vi "Previous Button Facade.vi"(0 "Data In":T4, 2 "Display State In":T2, 3 "Container State":T3) -> (6 "Data Out":T4, 7 "Display State Out":T2, 8 "Action":T1)   [LabVIEW 2010, in "Previous Button (System).xctl"]
uses:
  <vilib>/Navigation Controls/Previous Button System/Previous Button (System).xctl
  <vilib>/Navigation Controls/Previous Button System/Previous Button Data.ctl
  <vilib>/_xctls/Container State.ctl
  <vilib>/Navigation Controls/Previous Button System/Previous Button State.ctl
  <vilib>/_xctls/Action.ctl
  <vilib>/_xctls/XControlSupport.lvlib
  <vilib>/Navigation Controls/NI_Navigation.lvlib
panel:
  out "Error":bool
  in  "Prev Button":bool
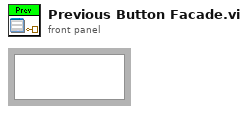
[diagram p1: front panel]
types:
  T1 = typedef "XControlSupport.lvlib/Action.ctl" = cluster{"Data Changed?":bool, "State Changed?":bool, "Action Name":string}
  T2 = typedef "Previous Button (System).xctl/Previous Button State.ctl" = cluster{"Button Text":string}
  T3 = typedef "XControlSupport.lvlib/Container State.ctl" = cluster{"Indicator?":bool, "Run Mode?":bool, " Refnum":refnum<vi>}
  T4 = typedef "Previous Button (System).xctl/Previous Button Data.ctl" = bool
  T5 = enum32{"Invalid", "Standard", "Closed", "Hidden", "Minimized", "Maximized"}
  T6 = enum32{"Bad", "Idle", "Run top level", "Running"}
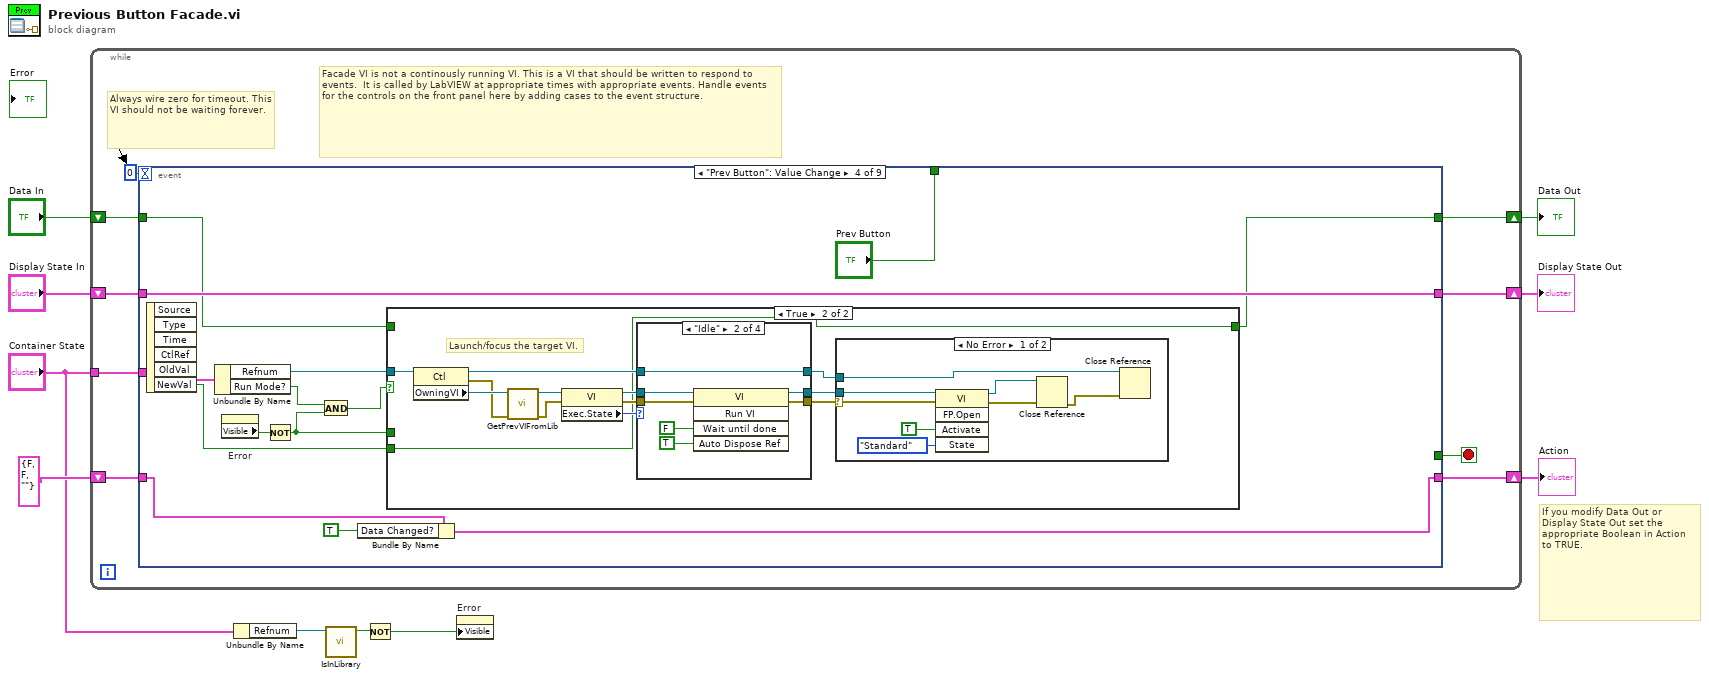
[diagram p0: block diagram]
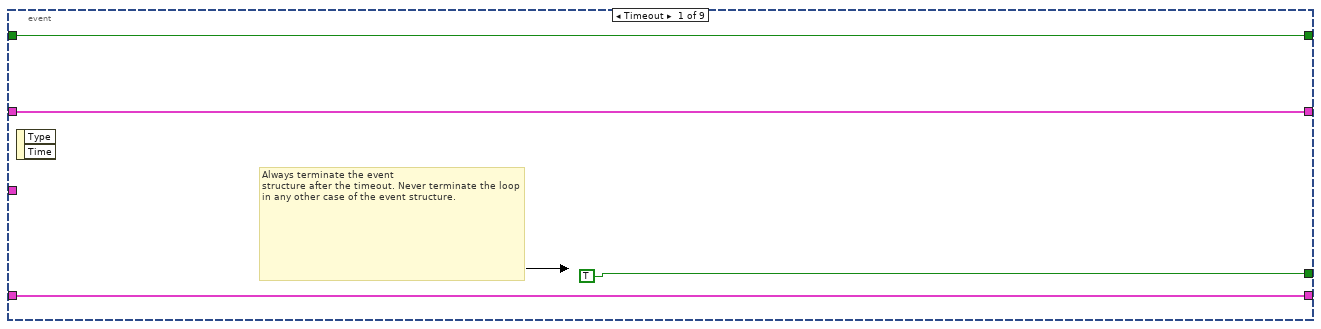
[diagram p2: hidden frame]
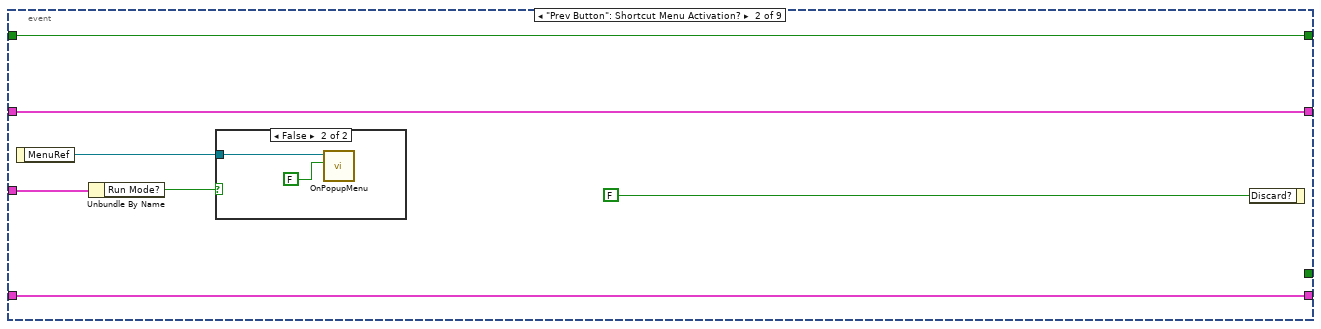
[diagram p3: hidden frame]
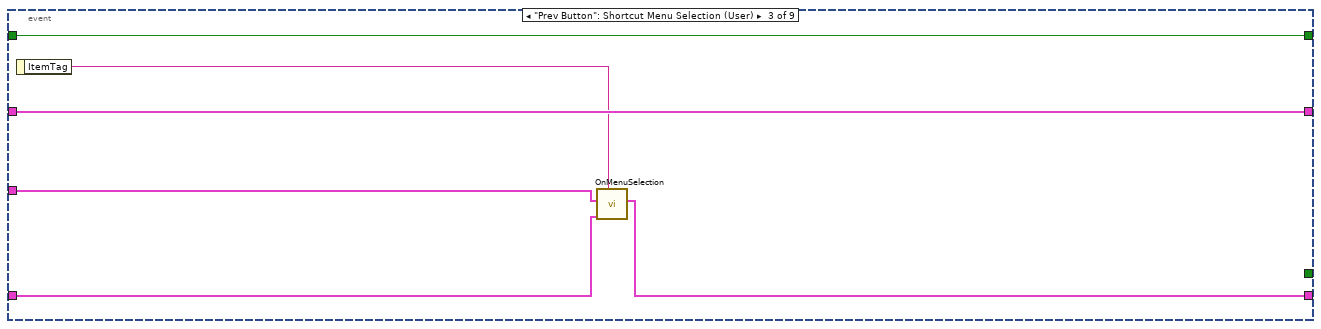
[diagram p5: hidden frame]
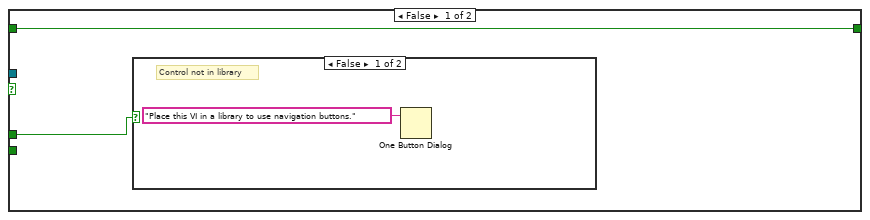
[diagram p6: hidden frame]
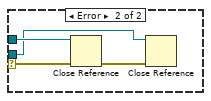
[diagram p8: hidden frame]
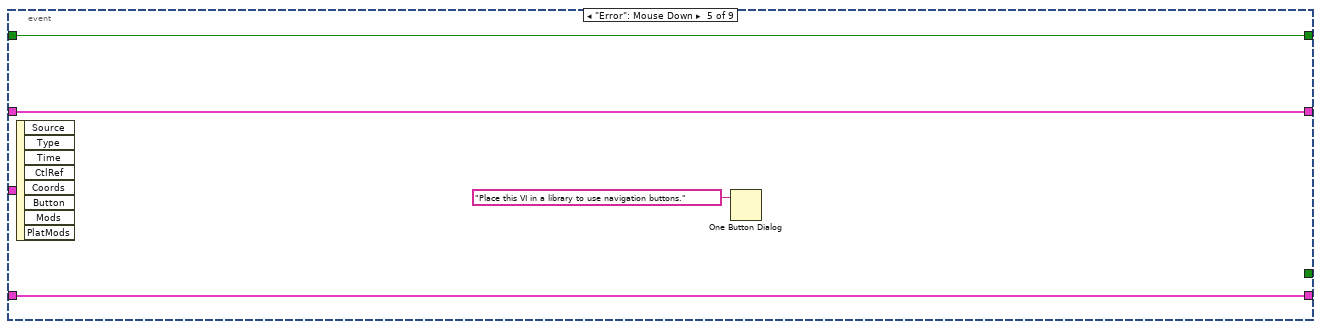
[diagram p12: hidden frame]
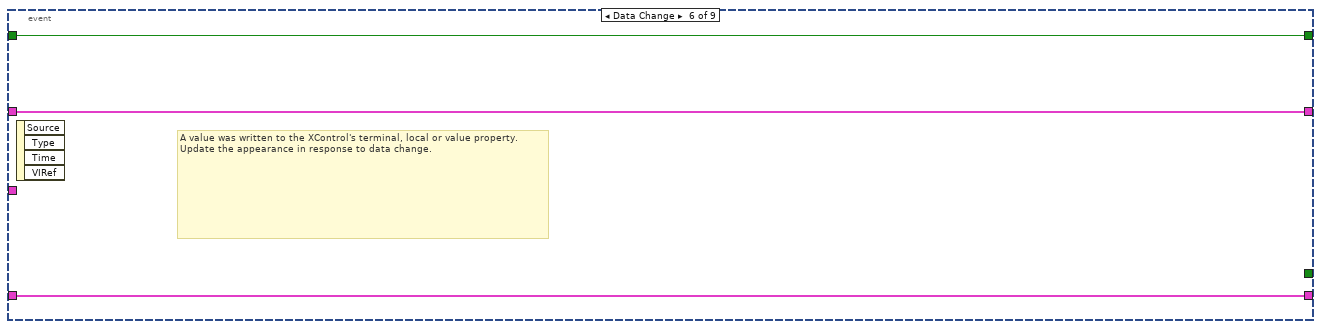
[diagram p13: hidden frame]
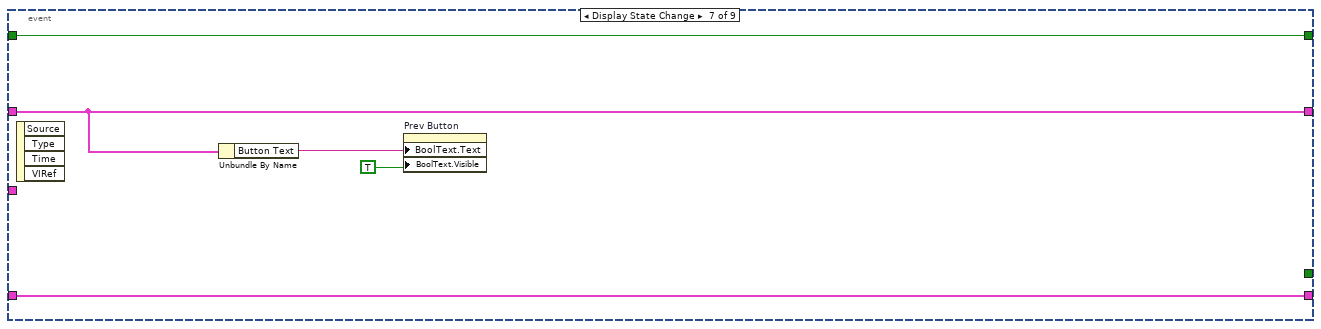
[diagram p14: hidden frame]
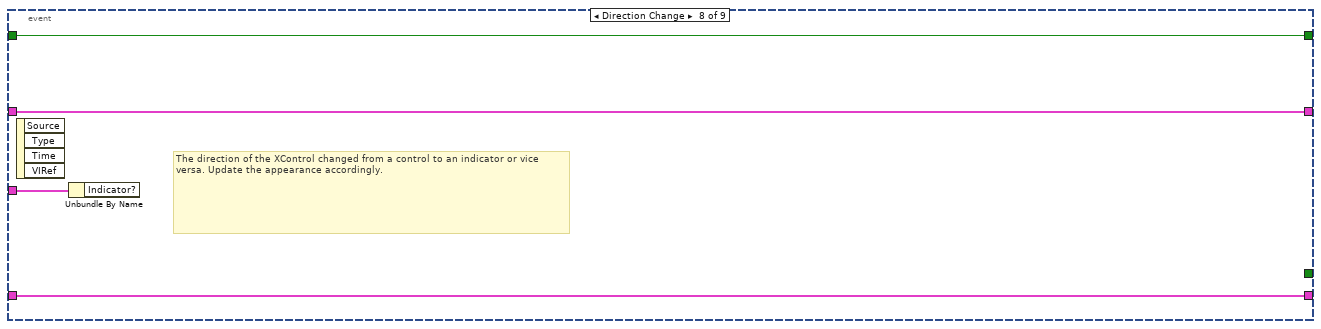
[diagram p15: hidden frame]
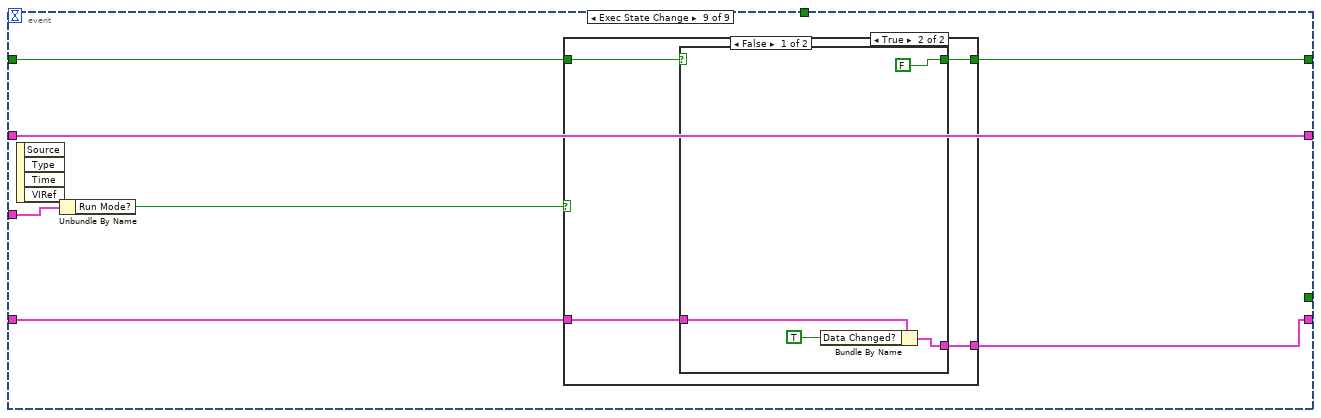
[diagram p16: hidden frame]
diagram:
  # "If you modify Data Out or\nDisplay State Out set the\nappropriate Boolean in Action\nto TRUE."
  n1 = while {
    shift-right: [w18] -> w8
    shift-left: "Display State In" -> [w19]
    tunnel: "Container State" -> [w15]
    shift-right: [w13] -> w10
    shift-left: "Data In" -> [w14]
    shift-right: [w11] -> w6
    shift-left: T1 {"Data Changed?"=FALSE, "State Changed?"=FALSE, "Action Name"=""} ("Action") -> [w12]
    stop <- w17 stop-if-true
    # "Facade VI is not a continously running VI. This is a VI that should be written to respond to events.  It is called by LabVIEW at appropriate times with appropriate events. Handle events for the controls on the front panel here by adding cases to the event structure."
    # "Always wire zero for timeout. This\nVI should not be waiting forever."
    n2 = event shown="[3] \"Prev Button\": Value Change" {
      selector: _ -> [_ _ _ _ _ _ _ _ _]
      dyn-events: _ -> [_ _ _ _ _ _ _ _ _]
      timeout: 0 -> [_ _ _ _ _ _ _ _ _]
      tunnel: w19 -> [w21 w29 w37 w52 w99 w102 w107 w111 w118]
      tunnel: [w21 w29 w37 w52 w99 w102 w107 w111 w118] -> w18
      tunnel: [TRUE _ _ _ _ _ _ _ _] -> w17
      tunnel: w15 -> [_ w27 w35 w48 _ _ _ w112 w119]
      tunnel: w14 -> [w20 w30 w38 w45 w100 w103 w108 w110 w116]
      tunnel: [w20 w30 w38 w43 w100 w103 w108 w110 w113] -> w13
      tunnel: [w22 w28 w33 w50 w98 w101 w106 w109 w115] -> w11
      tunnel: w12 -> [w22 w28 w36 w51 w98 w101 w106 w109 w117]
      tunnel: [_ _ _ "Prev Button" _ _ _ _ _] -> _
      event Timeout {
        # "Always terminate the event\nstructure after the timeout. Never terminate the loop in any other case of the event structure."
        n3 = event-data() -> ()  [unwired: 3 out]
      }
      event "Prev Button": Shortcut Menu Activation? {
        n4 = event-data() -> ("MenuRef"=w24:refnum<k9>)  [unwired: 1 out]
        n5 = Unbundle By Name(w27) -> ("Run Mode?"=w25:bool)
        n6 = case shown="False" w25 {
          tunnel: w24 -> [_ w32]
          frame True {
          }
          frame False {
            n7 = call <vilib>:"OnPopupMenu.vi"("Configurable?"=FALSE, "MenuRef"=w32) -> ()  [unwired: 10 in]
          }
        }
        n8 = event-data("Discard?"=FALSE) -> ()  [unwired: 1 in, 1 out]
      }
      event "Prev Button": Shortcut Menu Selection (User) {
        n9 = event-data() -> ("ItemTag"=w34:string)  [unwired: 1 out]
        n10 = call <vilib>:"OnMenuSelection.vi"("Tag"=w34, "Action In"=w36, "Container State"=w35) -> ("Action Out"=w33:T1)  [unwired: 7 in, 1 out]
      }
      event "Prev Button": Value Change {
        n11 = event-data() -> ("NewVal"=w44:bool)  [unwired: 6 out]
        n12 = Unbundle By Name(w48) -> ("Refnum"=w47:refnum<vi>, "Run Mode?"=w41:bool)
        n13 = property on="Error" class="Bool (strict)"() -> ("Visible"=w42:bool)  [unwired: 2 in, 2 out]
        n14 = Not(x=w42) -> (.not. x?=w39:bool)
        n15 = And(x=w41, y=w39) -> (x .and. y?=w40:bool)
        n16 = Bundle By Name(cluster=w51, "Data Changed?"=TRUE) -> (w50:T1)
        n17 = case shown="True" w40 {
          tunnel: w47 -> [_ w68]
          tunnel: w45 -> [w54 _]
          tunnel: w44 -> [_ w56]
          tunnel: [w54 w56] -> w43
          tunnel: w39 -> [w53 _]
          frame False {
            n18 = case shown="False" w53 {
              frame False {
                # "Control not in library"
                n19 = One Button Dialog(message="Place this VI in a library to use navigation buttons.") -> ()  [unwired: 2 out]
              }
              frame True {
                # "No problems"
              }
            }
          }
          frame True {
            # "Launch/focus the target VI."
            n20 = property class="Ctl"(reference=w68) -> (reference out=w58:refnum<vi>, error out=w66:errorcluster, "OwningVI"=w67:refnum<vi>)  [unwired: 1 in]
            n21 = call <vilib>:"GetPrevVIFromLib.vi"("error in (no error)"=w66, "VI Reference"=w67) -> ("error out"=w64:errorcluster, "Next VI"=w65:refnum<vi>)  [unwired: 8 out]
            n22 = property class="VI"(reference=w65, error in=w64) -> (reference out=w61:refnum<vi>, error out=w62:errorcluster, "Exec.State"=w63:T6)
            n23 = case shown="\"Idle\"" w63 {
              tunnel: w62 -> [w82 w90 w92 w96]
              tunnel: w61 -> [w83 w89 w93 w95]
              tunnel: [w82 w86 w92 w96] -> w59
              tunnel: [w83 w85 w93 w95] -> w60
              tunnel: w58 -> [w81 w84 w91 w94]
              tunnel: [w81 w84 w91 w94] -> w57
              frame "Bad", Default {
              }
              frame "Idle" {
                n24 = invoke class="VI" method="Run VI"(reference=w89, error in=w90, "Wait until done"=FALSE ("Wait Until Done"), "Auto Dispose Ref"=TRUE ("Auto Dispose Reference")) -> (reference out=w85:refnum<vi>, error out=w86:errorcluster)  [unwired: 1 in, 3 out]
              }
              frame "Run top level" {
              }
              frame "Running" {
              }
            }
            n25 = case shown="No Error" w59 {
              selector: w59 -> [w75 w79]
              tunnel: w60 -> [w76 w77]
              tunnel: w57 -> [w72 w80]
              frame No Error {
                n26 = invoke class="VI" method="FP.Open"(reference=w76, error in=w75, "Activate"=TRUE ("Activate?"), "State"=T5."Standard") -> (reference out=w71:refnum<vi>, error out=w70:errorcluster)  [unwired: 1 in, 3 out]
                n27 = Close Reference(reference=w71, error in (no error)=w70) -> (error out=w69:errorcluster)
                n28 = Close Reference(reference=w72, error in (no error)=w69) -> ()  [unwired: 1 out]
              }
              frame Error {
                n29 = Close Reference(reference=w80, error in (no error)=w79) -> (error out=w78:errorcluster)
                n30 = Close Reference(reference=w77, error in (no error)=w78) -> ()  [unwired: 1 out]
              }
            }
          }
        }
      }
      event "Error": Mouse Down {
        n31 = event-data() -> ()  [unwired: 9 out]
        n32 = One Button Dialog(message="Place this VI in a library to use navigation buttons.") -> ()  [unwired: 2 out]
      }
      event Data Change {
        # "A value was written to the XControl's terminal, local or value property.\nUpdate the appearance in response to data change."
        n33 = event-data() -> ()  [unwired: 5 out]
      }
      event Display State Change {
        n34 = event-data() -> ()  [unwired: 5 out]
        n35 = Unbundle By Name(w107) -> ("Button Text"=w105:string)
        n36 = property on="Prev Button" class="Bool"("BoolText.Text"=w105, "BoolText.Visible"=TRUE ("Boolean Text.Visible")) -> ()  [unwired: 2 in, 2 out]
      }
      event Direction Change {
        # "The direction of the XControl changed from a control to an indicator or vice versa. Update the appearance accordingly."
        n37 = event-data() -> ()  [unwired: 5 out]
        n38 = Unbundle By Name(w112) -> ()  [unwired: 1 out]
      }
      event Exec State Change {
        n39 = event-data() -> ()  [unwired: 5 out]
        n40 = Unbundle By Name(w119) -> ("Run Mode?"=w114:bool)
        n41 = case shown="False" w114 {
          tunnel: w117 -> [w123 w131]
          tunnel: [w122 w131] -> w115
          tunnel: w116 -> [w121 w130]
          tunnel: [w120 w130] -> w113
          frame False {
            n42 = case shown="True" w121 {
              selector: w121 -> [w124 _]
              tunnel: w123 -> [w125 w129]
              tunnel: [w125 w127] -> w122
              tunnel: [w124 T4 FALSE ("Data Out")] -> w120
              frame False {
              }
              frame True {
                n43 = Bundle By Name(cluster=w129, "Data Changed?"=TRUE) -> (w127:T1)
              }
            }
          }
          frame True {
          }
        }
      }
    }
  }
  "Display State Out" <- w8
  "Data Out" <- w10
  "Action" <- w6
  n44 = Unbundle By Name("Container State") -> ("Refnum"=w3:refnum<vi>)
  n45 = call <vilib>:"IsInLibrary.vi"("Control refnum"=w3) -> ("In library?"=w2:bool)  [unwired: 10 out]
  n46 = Not(x=w2) -> (.not. x?=w1:bool)
  n47 = property on="Error" class="Bool (strict)"("Visible"=w1) -> ()  [unwired: 2 in, 2 out]
